vi "Test Subtraction.vi"(8 "error in (no error)":errorcluster) -> (0 "error out":errorcluster)   [LabVIEW 2013]
doc: "This is an example test case."
uses:
  classes/Test/Test.lvclass
  classes/Assert/Assert.lvclass
panel:
  # "See block diagram"
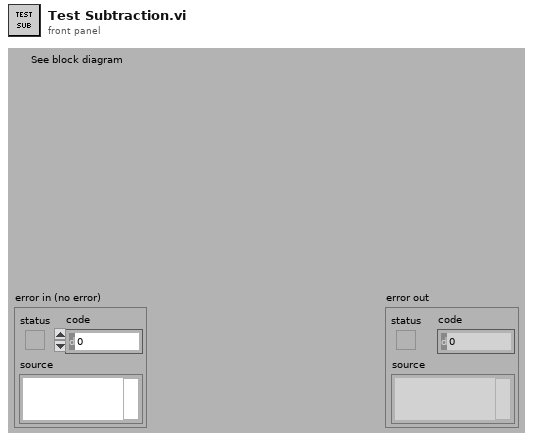
[diagram p1: front panel]
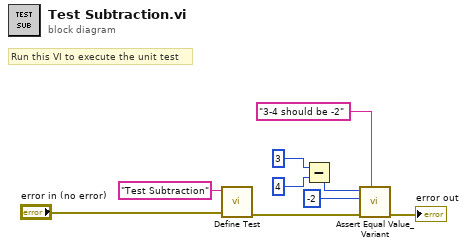
[diagram p0: block diagram]
diagram:
  # "Run this VI to execute the unit test"
  n1 = call "Define Test.vi"("error in (no error)"="error in (no error)", "Label (VI Title)"="Test Subtraction") -> ("error out"=w3:errorcluster)  [unwired: 9 in]
  n2 = Subtract(x=3, y=4) -> (x-y=w5:i32)
  n3 = call "Assert Equal Value_Variant.vi"("Label"="3-4 should be -2", "error in (no error)"=w3, "Y"=-2, "X"=w5) -> ("error out"=→"error out":errorcluster)  [unwired: 7 in]
